vi "Test Line Intersection With Sprite 2.vi"(11 "Test Case In":refnum<class "Collision Tests.lvclass">) -> (3 "Test Case Out":refnum<class "Collision Tests.lvclass">)   [LabVIEW 2021, in "Collision Tests.lvclass"]
uses:
  Collision Tests.lvclass
  C:/Program Files (x86)/National Instruments/LabVIEW 2026/vi.lib/Astemes/LUnit/Test Case.lvclass
  Re-use Libraries/Vector 2D/Vector 2D.lvclass
  <vilib>/Astemes/LUnit/Test Case.lvclass/Test Case.ctl
  Collision Tests.lvclass/Collision Tests.ctl
  Re-use Libraries/Collision/Collision.lvlib
  Re-use Libraries/Utility/Utility.lvlib
  90291e97-5563-4cfe-8842-a806efdb4406.vi
  <vilib>/Astemes/LUnit/Test Case.lvclass
  Re-use Libraries/Utility/Typedef/Line.ctl
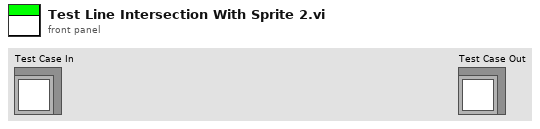
[diagram p1: front panel]
types:
  T1 = typedef "Utility.lvlib/Line.ctl" = cluster{"Start Point":refnum<class "Vector 2D.lvclass">, "End Point":refnum<class "Vector 2D.lvclass">}
  T2 = typedef "imagedata.ctl" = cluster{"image type":i32, "image depth":i32, "image":u8[], "mask":u8[], "colors":u32[], "Rectangle":cluster{"left":i16, "top":i16, "right":i16, "bottom":i16}}
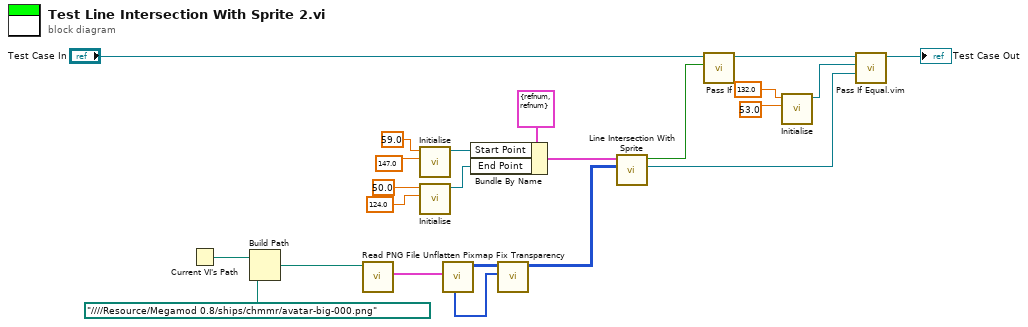
[diagram p0: block diagram]
diagram:
  n1 = Current VI's Path() -> (path=w23:path)
  n2 = Build Path(base path=w23, name or relative path=path "../../../../Resource/Megamod 0.8/ships/chmmr/avatar-big-000.png" ("Path")) -> (appended path=w21:path)
  n3 = call <vilib>:"Read PNG File.vi"("path to PNG file"=w21) -> ("image data"=w20:T2)  [unwired: 8 in, 2 out]
  n4 = call "Initialise.vi"("y"=sgl 147.0 ("x"), "x"=sgl 59.0) -> ("Vector 2D out"=w6:refnum<class "Vector 2D.lvclass">)  [unwired: 9 in]
  n5 = call "Initialise.vi"("y"=sgl 124.0 ("x"), "x"=sgl 50.0) -> ("Vector 2D out"=w5:refnum<class "Vector 2D.lvclass">)  [unwired: 9 in]
  n6 = call <vilib>:"Unflatten Pixmap.vi"("image data"=w20) -> ("24-bit pixmap"=w18:u32[][], "mask"=w19:u8[])  [unwired: 4 in, 5 out]
  n7 = Bundle By Name(cluster=T1 {"Start Point"=refnum, "End Point"=refnum} ("Line"), "Start Point"=w6, "End Point"=w5) -> (w1:T1)
  n8 = call "Fix Transparency.vi"("Mask"=w19, "Pixels In"=w18) -> ("Pixels Out"=w2:u32[][])  [unwired: 9 in]
  n9 = call "Line Intersection With Sprite.vi"("Pixel Data in"=w2, "Line"=w1) -> ("Hit Point"=w13:refnum<class "Vector 2D.lvclass">, "Hit"=w14:bool)  [unwired: 8 in]
  n10 = call <vilib>:"Pass If.vi"("Pass?"=w14, "LUnit Test Case In"="Test Case In") -> ("LUnit Test Case Out"=w15:refnum<class "Collision Tests.lvclass">)  [unwired: 8 in, 1 out]
  n11 = call "Initialise.vi"("y"=sgl 53.0 ("x"), "x"=sgl 132.0) -> ("Vector 2D out"=w10:refnum<class "Vector 2D.lvclass">)  [unwired: 9 in]
  n12 = call "Pass If Equal.vim"("Actual"=w13, "Expected"=w10, "LUnit Test Case In"=w15) -> ("LUnit Test Case Out"=→"Test Case Out":refnum<class "Collision Tests.lvclass">)  [unwired: 7 in, 1 out]
